vi "AvrgDBL.vi"(4 "b":dbl, 5 "a":dbl) -> (1 "Average of a and b":dbl)   [LabVIEW 2017, in "GPNumeric.lvlib"]
doc: "Calculates the average value of <B>a</B> and <B>b</B>.\n\nThis VI is inlined.\n\nSteen Schmidt\nGPower\n24/11 2014"
uses:
  GPNumeric.lvlib
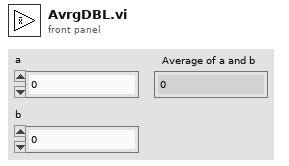
[diagram p1: front panel]
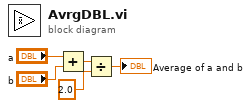
[diagram p0: block diagram]
diagram:
  n1 = Add(x="a", y="b") -> (x+y=w3:dbl)
  n2 = Divide(x=w3, y=2.0) -> (x/y=→"Average of a and b":dbl)
